vi "定时设置写入.vi"(10 "INI Fomatted Cluster":variant, 11 "测试参数":string) -> ()   [LabVIEW 2016, in "定时设置.xctl"]
uses:
  <vilib>/Utility/config.llb/NI_LVConfig.lvlib
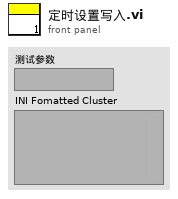
[diagram p1: front panel]
types:
  T1 = typedef "NI_LVConfig.lvlib/Config Data RefNum.ctl" = refnum<k1>
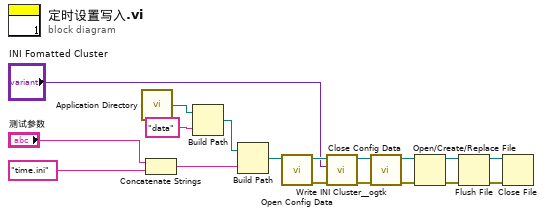
[diagram p0: block diagram]
diagram:
  n1 = call <vilib>:"Application Directory.vi"() -> ("Application Directory"=w18:path)
  n2 = Concatenate Strings("测试参数", "time.ini" ("名称或相对路径")) -> (w4:string)
  n3 = Build Path(base path=w18, name or relative path="data" ("名称或相对路径")) -> (appended path=w6:path)
  n4 = Build Path(base path=w6, name or relative path=w4) -> (appended path=w2:path)
  n5 = call <vilib>:"Open Config Data.vi"("configuration file path"=w2) -> ("error out"=w15:errorcluster, "refnum"=w17:T1)  [unwired: 8 in, 1 out]
  n6 = call <userlib>:"Write INI Cluster__ogtk.vi"("error in (no error)"=w15, "INI Fomatted Cluster"="INI Fomatted Cluster", "refnum"=w17) -> ("error out"=w14:errorcluster, "dup refnum"=w16:T1)  [unwired: 7 in]
  n7 = call <vilib>:"Close Config Data.vi"("error in (no error)"=w14, "refnum"=w16) -> ("error out"=w9:errorcluster, "file path"=w8:path)  [unwired: 8 in]
  n8 = Open/Create/Replace File(file path (use dialog)=w8, error in=w9) -> (refnum out=w12:refnum<file>, error out=w13:errorcluster)  [unwired: 4 in, 1 out]
  n9 = Flush File(refnum=w12, error in=w13) -> (refnum out=w11:refnum<file>, error out=w10:errorcluster)
  n10 = Close File(refnum=w11, error in=w10) -> ()  [unwired: 2 out]
